vi "NTV_AutoRIO String.vi"(7 "Read(f) Write(t)":bool, 11 "Auto RIO":string) -> (3 "Auto RIO":string)   [LabVIEW 2023]
uses:
  <vilib>/Rock Robotics/Network Tables/NT Read String.vi
  <vilib>/Rock Robotics/Network Tables/NT Write String.vi
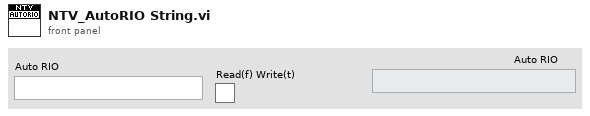
[diagram p1: front panel]
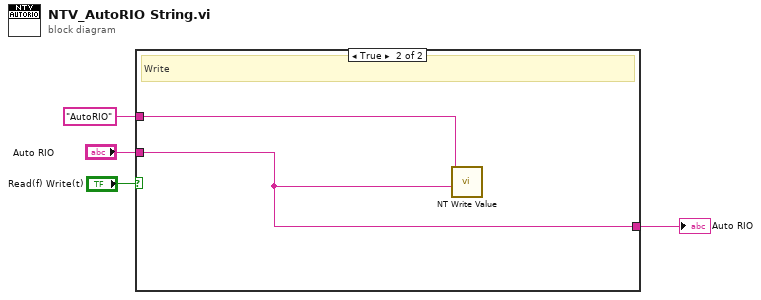
[diagram p0: block diagram]
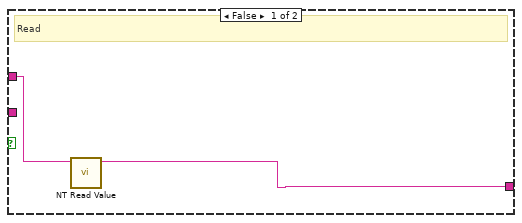
[diagram p2: hidden frame]
diagram:
  n1 = case shown="True" "Read(f) Write(t)" {
    tunnel: "AutoRIO" ("Name") -> [w6 w8]
    tunnel: [w5 w7] -> w2
    tunnel: "Auto RIO" -> [_ w7]
    frame False {
      # "Read"
      n2 = call-poly <vilib>:"NT Read Value.vi"("name"=w6) -> ("value"=w5:string)  [unwired: 8 in, 2 out]
    }
    frame True {
      # "Write"
      n3 = call-poly <vilib>:"NT Write Value.vi"("value"=w7, "name"=w8) -> ()  [unwired: 9 in, 1 out]
    }
  }
  "Auto RIO" <- w2
